vi "Run_Powershell_script.vi"(8 "error in":errorcluster, 11 "Powershell Script":string="$file = \"C:\\Users\\monke\\Desktop\\Work\\VIs to modify\\ONENOTE\\Sandbox\\curl-logo.jpg\"\n\n$read = [convert]::ToBase64String((Get-Content $file -Encoding byte))\n$imageDataURL = [string]::Format(\"data:image/jpeg;base64,{0}\", $read)\n\n$requestBodyPrefix = @\"\n--BlockBoundary\nContent-Disposition:form-data; name=\"Commands\"\nContent-Type:application/json\n\n[{\n\t\"target\": \"body\",\n\t\"action\": \"append\",\n    \"content\": \"<img src=\n\"@\n$requestBodySuffix = @\"\n alt='There is something wrong with the request or the rendering. Please contact Joe'/>\"\n}]\n\n\n--BlockBoundary--\n\"@\n$request1 = $requestBodyPrefix + $imageDataUrl\n$request1 = $request1 + $requestBodySuffix\n$url = 'https://www.onenote.com/api/v1.0/me/notes/pages/0-c8e01dcaf69a4df09e4cc94142adbb9e!47-962DFAE583894FEA!201/content'\n$AccessToken = \"EwAQA61DBAAUcSSzoTJJsy+XrnQXgAKO5cj4yc8AAS6fPc6NVokthrh8Aw3FulD0hYgp7aZyj/mtVLeNARi4RLEL0/Wbr+rQ+0AvAsSRTkAWVMDQenSKh3916rQ85Gi3BaxeKzlXgS3hIOzsyXteoja2swX0Yy/1ucSuS3PDQsNsc6D+dlzpkERiGEPaEM4C//uC08x5ROEVfkqO5qsj9vHtLbpX0ZCKsVCARpgHh/v8EAZ75OQw0wYmVfsnL9pZBkDMYtv+GoWXPRQmR+2Sd7ty0WQ7JFfFKhLPOdTk5IUBzl1KymiBFBgS9/xeWrV0a0XDjUhSpU4molMTKc/7WwM//43cHjzl8+78h4u54CKg21krOqq9f+r7Wj7+KCEDZgAACBFzrI8vXCWb4AGpj4eW2Lohr6Sce8fSAOXqdJUoNi3c03rx/WjvC8HM0K6iV2pp6ODZw2KkXuwMYr1knYE0MKapS2g5jz9CrfvzlP2IFeJrBZMUFsOZMxDYAGs4VPi+ipBSFiX69l16fsZ7e12QBUwcLFCUGZ8x2B/Lvcn8lxNKLhEiPQZyEPufenBbV1NrXOV3uGrJLnypB/BtSZMXIrzFw1zf3mhjKVlKE60mqBBx2ackS+a1LElmOASeBc5IsWqshnYxDx6Hslk910n9RbW0iJZXq5acSUqrxrFIkL1nQlqaeVLaAOUYZBhWDMf7Yzw0/xmUVWAyNHpbud+ZUnDnqpf50evEFonPML6fdW0j+1tVMlltMBvVGTZhy7S3UYrWEmmFAi8ET9mm7AtAc1M9rkCdg6uWeDUeb3ydVOJuExCN5rarazj6+Akimov2ol+wPBWL8NLKzHNpS0c9FTQxypnvwGHenvEnOM78Zl4/IgorEos1yHjfGAkSXp2d7QsT9xf+Xba6PbWCfdRvPekCM+6niRDMjU4Eh9kwLdFxilBQRoxF1lEmcg7EAEOMG71Shz/N/SbI+ti0UdK83MN1keRzMkK5hEiNfSd6YfPLQv39MOg60CcCkbLD779TWLQd8k0otHQ5YnMWAg==\"\n$headers = @{\"Authorization\" = \"Bearer \" + $AccessToken}\n\nInvoke-RestMethod -method 'PATCH' -uri $url -Body $request1 -Headers $headers -ContentType 'multipart/form-data; boundary=BlockBoundary'") -> (0 "error out":errorcluster, 2 "standard error":string, 3 "standard output":string)   [LabVIEW 2016]
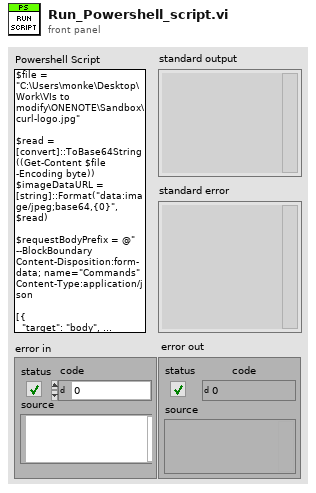
[diagram p1: front panel]
types:
  T1 = enum16{"open", "replace", "create", "open or create", "replace or create", "replace or create with confirmation"}
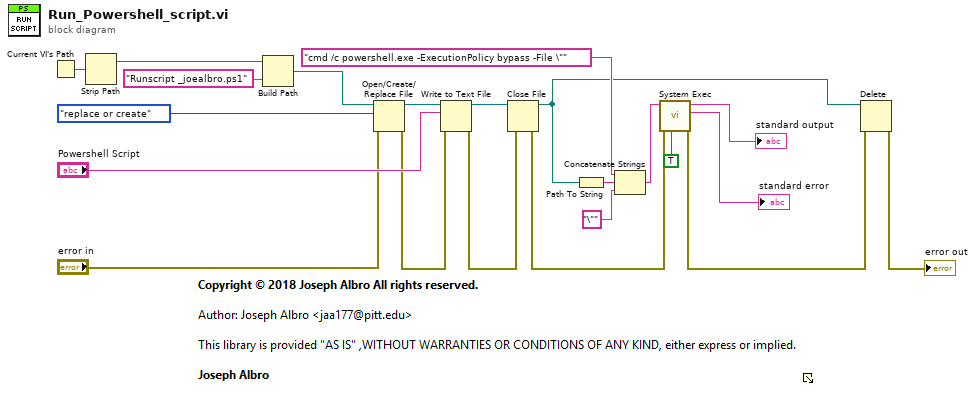
[diagram p0: block diagram]
diagram:
  n1 = Current VI's Path() -> (path=w5:path)
  n2 = Strip Path(path=w5) -> (stripped path=w4:path)  [unwired: 1 out]
  n3 = Build Path(base path=w4, name or relative path="Runscript _joealbro.ps1" ("string")) -> (appended path=w2:path)
  n4 = Open/Create/Replace File(file path (use dialog)=w2, error in="error in", operation (0:open)=T1."replace or create") -> (refnum out=w14:refnum<file>, error out=w12:errorcluster)  [unwired: 3 in, 1 out]
  n5 = Write to Text File(file (use dialog)=w14, text="Powershell Script", error in=w12) -> (refnum out=w13:refnum<file>, error out=w11:errorcluster)  [unwired: 1 in, 1 out]
  n6 = Close File(refnum=w13, error in=w11) -> (path=w1:path, error out=w10:errorcluster)
  n7 = Path To String(path=w1) -> (string=w17:string)
  n8 = Concatenate Strings("cmd /c powershell.exe -ExecutionPolicy bypass -File \"" ("command line"), w17, "\"" ("string")) -> (w16:string)
  n9 = call <vilib>:"System Exec.vi"("run minimized? (F)"=TRUE, "error in (no error)"=w10, "command line"=w16) -> ("error out"=w8:errorcluster, "standard error"=→"standard error":string, "standard output"=→"standard output":string)  [unwired: 5 in, 1 out]
  n10 = Delete(path (use dialog)=w1, error in=w8) -> (error out=→"error out":errorcluster)  [unwired: 3 in, 2 out]
